vi "dfd_PR Cosine-Modulated Generate Coefficients.vi"(10 "M":i32, 11 "phi":dbl[](array[numeric])) -> (3 "p":dbl[](array[numeric]))   [LabVIEW 2017, in "NI_DigFilter_FilterBank.lvlib"]
uses:
  <vilib>/addons/Digital Filter Design/NI_DigFilter_FilterBank.lvlib
  <vilib>/Analysis/baseanly.llb/Real A x B.vi
  <vilib>/Analysis/7linalg.llb/Real Transpose Matrix.vi
  <vilib>/Analysis/NI_AALPro.lvlib
  <vilib>/Analysis/NI_AALBase.lvlib
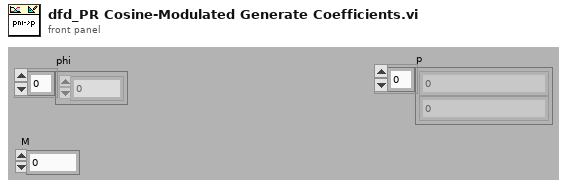
[diagram p1: front panel]
types:
  T1 = typedef "NI_Matrix.lvlib/RealMatrix.ctl" = dbl[][]
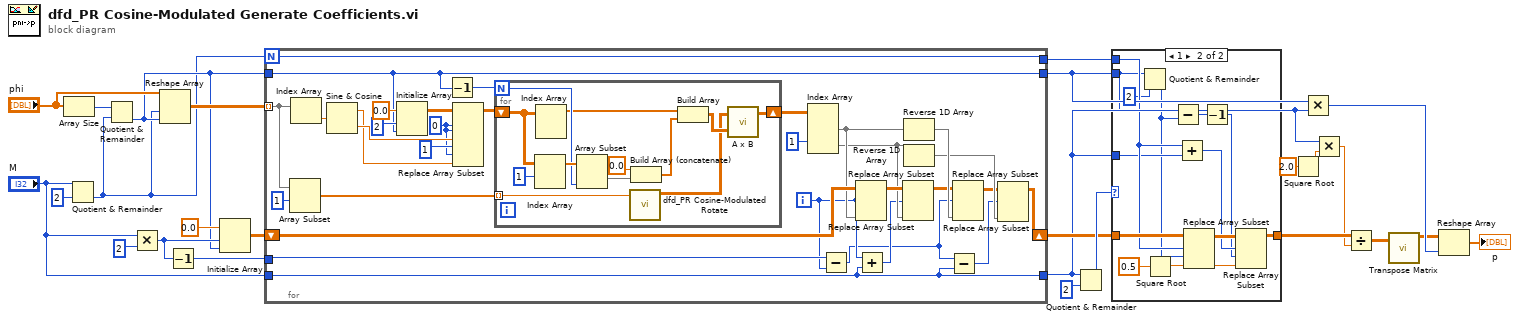
[diagram p0: block diagram]
diagram:
  n1 = Array Size(array="phi") -> (size(s)=w25:i32)
  n2 = Quotient & Remainder(x="M", y=2) -> (floor(x/y)=w10:i32)  [unwired: 1 out]
  n3 = Quotient & Remainder(x=w25, y=w10) -> (floor(x/y)=w11:i32)  [unwired: 1 out]
  n4 = Multiply(x="M", y=2) -> (x*y=w19:i32)
  n5 = Reshape Array("phi", w10, w11) -> (w12:dbl[][])
  n6 = Decrement(x=w19) -> (x-1=w18:i32)
  n7 = Initialize Array(0.0 ("element"), w19, w11) -> (w21:dbl[][])
  n8 = for {
    N: w10 -> [w33]
    tunnel: w12 -> [w50] mode=indexing
    tunnel: w11 -> [w29]
    shift-right: [w27] -> w15
    shift-left: w21 -> [w45]
    tunnel: "M" -> [w34]
    tunnel: w18 -> [w41]
    tunnel: [w34] -> w5
    tunnel: [w33] -> w14
    tunnel: [w29] -> w13
    i -> [w40]
    w53 = 0 ("index (row)")
    n9 = Array Subset(array=w50, index=1) -> (w48:dbl[])  [unwired: 1 in]
    n10 = Index Array(array=w50) -> (element=w51:dbl)  [unwired: 1 in]
    n11 = Sine & Cosine(0:w51) -> (1:w52:dbl, 2:w54:dbl)
    n12 = Initialize Array(0.0 ("element"), 2 ("dimension size"), w29) -> (w56:dbl[][])
    n13 = Decrement(x=w29) -> (x-1=w28:i32)
    n14 = Replace Array Subset(array=w56, new element #1=w54, index (row) #1=w53, index (col) #1=w53, new element #2=w52, index (row) #2=1 ("index (row)"), index (col) #2=w53) -> (w30:dbl[][])
    n15 = for {
      N: w28 -> [w68]
      shift-right: [w62] -> w47
      shift-left: w30 -> [w65]
      tunnel: w48 -> [w63] mode=indexing
      n16 = Index Array(array=w65, index (row)=1) -> (element=w69:dbl[])  [unwired: 1 in]
      n17 = Index Array(array=w65) -> (element=w64:dbl[])  [unwired: 2 in]
      n18 = Array Subset(array=w69, length=w68) -> (w67:dbl[])  [unwired: 1 in]
      n19 = call <vilib>:"dfd_PR Cosine-Modulated Rotate.vi"("angle"=w63) -> ("rotate"=w60:dbl[][])  [unwired: 10 in]
      n20 = Build Array (concatenate)(0.0, w67) -> (w59:dbl[])
      n21 = Build Array(w64, w59) -> (w61:dbl[][])
      n22 = call-poly <vilib>:"A x B.vi"("B"=w61, "A"=w60) -> ("A x B"=w62:T1)  [unwired: 1 out]
    }
    n23 = Index Array(array=w47, index (row) #2=1 ("index (row)")) -> (element #1=w43:dbl[], element #2=w42:dbl[])  [unwired: 3 in]
    n24 = Subtract(x=w41, y=w40) -> (x-y=w36:i32)
    n25 = Replace Array Subset(array=w45, new element=w43, index (row)=w40) -> (w44:dbl[][])  [unwired: 1 in]
    n26 = Add(x=w40, y=w34) -> (x+y=w39:i32)
    n27 = Replace Array Subset(array=w44, new element=w42, index (row)=w39) -> (w31:dbl[][])  [unwired: 1 in]
    n28 = Reverse 1D Array(array=w43) -> (reversed array=w38:dbl[])
    n29 = Reverse 1D Array(array=w42) -> (reversed array=w37:dbl[])
    n30 = Subtract(x=w36, y=w34) -> (x-y=w35:i32)
    n31 = Replace Array Subset(array=w31, new element=w38, index (row)=w36) -> (w32:dbl[][])  [unwired: 1 in]
    n32 = Replace Array Subset(array=w32, new element=w37, index (row)=w35) -> (w27:dbl[][])  [unwired: 1 in]
  }
  n33 = Quotient & Remainder(x=w5, y=2) -> (x-y*floor(x/y)=w16:i32)  [unwired: 1 out]
  n34 = case shown="1" w16 {
    tunnel: w15 -> [w71 w84]
    tunnel: [w71 w78] -> w8
    tunnel: w13 -> [_ w76]
    tunnel: w14 -> [_ w81]
    tunnel: w5 -> [_ w80]
    frame 0, Default {
    }
    frame 1 {
      n35 = Quotient & Remainder(x=w76, y=2) -> (floor(x/y)=w75:i32)  [unwired: 1 out]
      n36 = Square Root(x=0.5) -> (sqrt(x)=w72:dbl)
      n37 = Subtract(x=w76, y=w75) -> (x-y=w74:i32)
      n38 = Add(x=w81, y=w80) -> (x+y=w79:i32)
      n39 = Replace Array Subset(array=w84, new element=w72, index (row)=w81, index (col)=w75) -> (w82:dbl[][])
      n40 = Decrement(x=w74) -> (x-1=w73:i32)
      n41 = Replace Array Subset(array=w82, new element=w72, index (row)=w79, index (col)=w73) -> (w78:dbl[][])
    }
  }
  n42 = Square Root(x=2.0) -> (sqrt(x)=w2:dbl)
  n43 = Multiply(x=w13, y=w5) -> (x*y=w9:i32)
  n44 = Multiply(x=w5, y=w2) -> (x*y=w4:dbl)
  n45 = Divide(x=w8, y=w4) -> (x/y=w1:dbl[][])
  n46 = call-poly <vilib>:"Transpose Matrix.vi"("Input Matrix"=w1) -> ("Matrix Transpose"=w7:T1)  [unwired: 9 in, 1 out]
  n47 = Reshape Array(w7, w9) -> (→"p":dbl[])
